vi "Check Reference Type.vi"(8 "error in (no error)":errorcluster, 11 "Refnum Value Source in":refnum<class "Ctrl Refnum Value Source.lvclass">) -> (0 "error out":errorcluster, 3 "Refnum Value Source out":refnum<class "Ctrl Refnum Value Source.lvclass">)   [LabVIEW 2020, in "Composed Columns.lvlib" / "Ctrl Refnum Value Source.lvclass"]
uses:
  Ctrl Refnum Value Source.lvclass
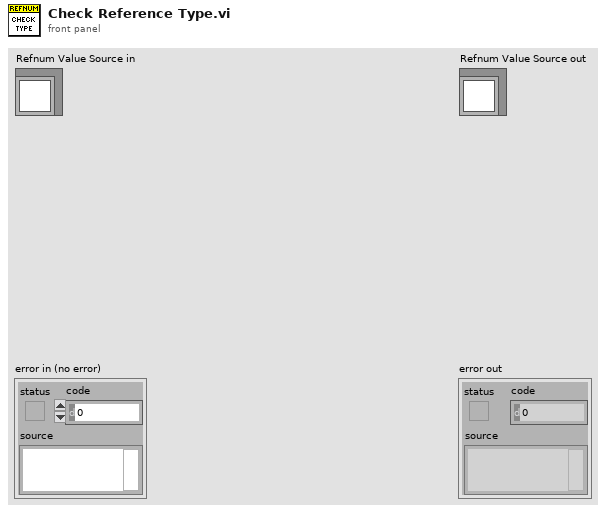
[diagram p1: front panel]
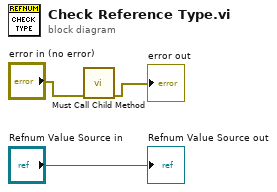
[diagram p0: block diagram]
diagram:
  n1 = call "Must Call Child Method.vi"("error in"="error in (no error)") -> ("error out"=→"error out":errorcluster)  [unwired: 10 in]
  "Refnum Value Source out" <- "Refnum Value Source in"
